vi "save_column_width.vi"(8 "error in (no error)":errorcluster, 11 "listbox_reference":refnum<vi>) -> (0 "error out":errorcluster, 2 "configuration []":cluster{"width":u32, "height":u32}[](array[cluster]))   [LabVIEW 2015, in "lv-pagination.lvlib"]
uses:
  lv-pagination.lvlib
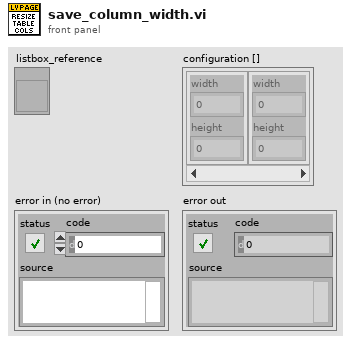
[diagram p1: front panel]
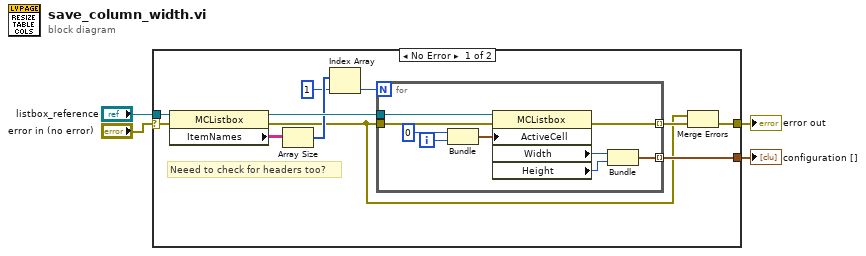
[diagram p0: block diagram]
diagram:
  n1 = case shown="No Error" "error in (no error)" {
    selector: "error in (no error)" -> [w15 w25]
    tunnel: "listbox_reference" -> [w7 _]
    tunnel: [w13 w25] -> w3
    tunnel: [w8 _] -> w2
    frame No Error {
      # "Neeed to check for headers too?"
      n2 = property on="Property Node" class="MCListbox"(reference=w7, error in=w15) -> (reference out=w11:refnum<vi>, error out=w5:errorcluster, "ItemNames"=w12:string[][])
      n3 = Array Size(array=w12) -> (size(s)=w10:i32[])
      n4 = Index Array(array=w10, index=1) -> (element=w9:i32)
      n5 = for {
        N: w9 -> [_]
        tunnel: w11 -> [w24]
        tunnel: [w23] -> w14 mode=indexing
        tunnel: w5 -> [w21]
        tunnel: [w16] -> w8 mode=indexing
        i -> [w20]
        n6 = Bundle("Column"=0, w20) -> (w22:cluster{"Column":i32, i32})  [unwired: 1 in]
        n7 = property on="Property Node" class="MCListbox"(reference=w24, error in=w21, "ActiveCell"=w22) -> (error out=w23:errorcluster, "Width"=w18:u32, "Height"=w17:u32)  [unwired: 1 out]
        n8 = Bundle("Width"=w18, "Height"=w17) -> (w16:cluster{"Width":u32, "Height":u32})  [unwired: 1 in]
      }
      n9 = Merge Errors(w5, w14) -> (w13:errorcluster)
    }
    frame Error {
    }
  }
  "error out" <- w3
  "configuration []" <- w2
